vi "Get Joint Position.vi"(6 "JointType":T2 items=["SpineBase", "SpineMid", "Neck", "Head", "ShoulderLeft", "ElbowLeft", "WristLeft", "HandLeft", "ShoulderRight", "ElbowRight", "WristRight", "HandRight", "HipLeft", "KneeLeft", "AnkleLeft", "FootLeft", "HipRight", "KneeRight", "AnkleRight", "FootRight", "SpineShoulder", "HandTipLeft", "ThumbLeft", "HandTipRight", "ThumbRight"], 8 "error in (no error)":errorcluster, 9 "Coordinate Space":enum16{"Color Space", "Depth Space"}(ring), 10 "Joints":refnum<k24>, 11 "KinectSensor Reference":refnum<k24>) -> (0 "error out":errorcluster, 3 "Joint Position":T1 {"TrackingState" items=["NotTracked", "Inferred", "Tracked"]})   [LabVIEW 2014]
uses:
  Microsoft.Kinect
  controls/JointType.ctl
  controls/Joint Position.ctl
  Constants.vi
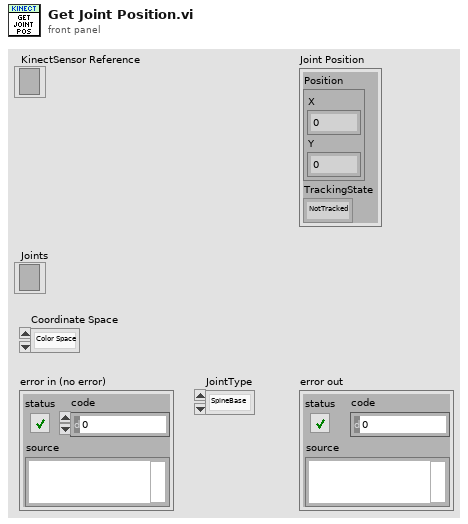
[diagram p1: front panel]
types:
  T1 = typedef "Joint Position.ctl" = cluster{"Position":cluster{"X":sgl, "Y":sgl}, "TrackingState":i32}
  T2 = typedef "JointType.ctl" = i32
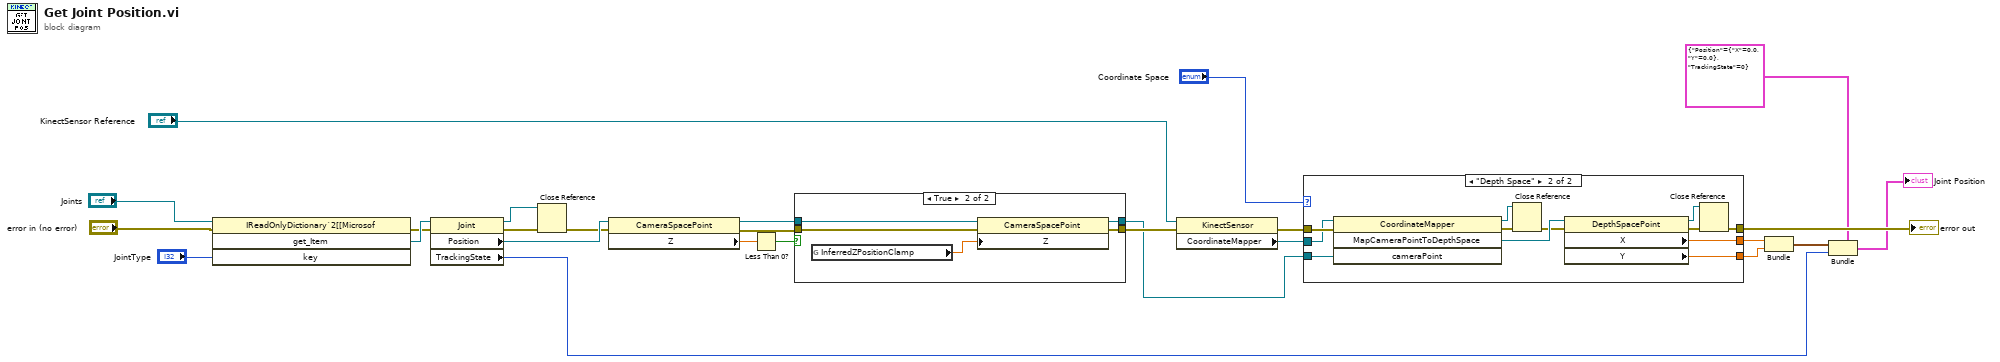
[diagram p0: block diagram]
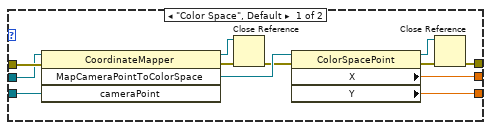
[diagram p2: hidden frame]
diagram:
  n1 = invoke class="IReadOnlyDictionary`2[[Microsof" method="get_Item"(reference="Joints", error in="error in (no error)", "key"="JointType") -> (error out=w13:errorcluster, "get_Item"=w14:refnum<k24>)  [unwired: 1 in, 2 out]
  n2 = property class="Joint"(reference=w14, error in=w13) -> (reference out=w8:refnum<k24>, error out=w9:errorcluster, "Position"=w12:refnum<k24>, "TrackingState"=w3:i32)
  n3 = Close Reference(reference=w8, error in (no error)=w9) -> (error out=w7:errorcluster)
  n4 = property class="CameraSpacePoint"(reference=w12, error in=w7) -> (reference out=w21:refnum<k24>, error out=w20:errorcluster, "Z"=w23:sgl)
  n5 = Less Than 0?(x=w23) -> (x < 0?=w22:bool)
  n6 = case shown="True" w22 {
    tunnel: w21 -> [w27 w32]
    tunnel: w20 -> [w28 w31]
    tunnel: [w28 w30] -> w19
    tunnel: [w27 w29] -> w18
    frame False {
    }
    frame True {
      n7 = global read "Constants.vi" "InferredZPositionClamp"() -> (w33:sgl)
      n8 = property class="CameraSpacePoint"(reference=w32, error in=w31, "Z"=w33) -> (reference out=w29:refnum<k24>, error out=w30:errorcluster)
    }
  }
  n9 = property class="KinectSensor"(reference="KinectSensor Reference", error in=w19) -> (error out=w26:errorcluster, "CoordinateMapper"=w25:refnum<k24>)  [unwired: 1 out]
  n10 = case shown="\"Depth Space\"" "Coordinate Space" {
    tunnel: w26 -> [w45 w57]
    tunnel: w25 -> [w44 w56]
    tunnel: w18 -> [w43 w55]
    tunnel: [w41 w53] -> w17
    tunnel: [w40 w52] -> w16
    tunnel: [w34 w46] -> w5
    frame "Color Space", Default {
      n11 = invoke class="CoordinateMapper" method="MapCameraPointToColorSpace"(reference=w44, error in=w45, "cameraPoint"=w43) -> (reference out=w37:refnum<k24>, error out=w39:errorcluster, "MapCameraPointToColorSpace"=w42:refnum<k24>)  [unwired: 1 in, 1 out]
      n12 = Close Reference(reference=w37, error in (no error)=w39) -> (error out=w38:errorcluster)
      n13 = property class="ColorSpacePoint"(reference=w42, error in=w38) -> (reference out=w35:refnum<k24>, error out=w36:errorcluster, "X"=w40:sgl, "Y"=w41:sgl)
      n14 = Close Reference(reference=w35, error in (no error)=w36) -> (error out=w34:errorcluster)
    }
    frame "Depth Space" {
      n15 = invoke class="CoordinateMapper" method="MapCameraPointToDepthSpace"(reference=w56, error in=w57, "cameraPoint"=w55) -> (reference out=w49:refnum<k24>, error out=w51:errorcluster, "MapCameraPointToDepthSpace"=w54:refnum<k24>)  [unwired: 1 in, 1 out]
      n16 = Close Reference(reference=w49, error in (no error)=w51) -> (error out=w50:errorcluster)
      n17 = property class="DepthSpacePoint"(reference=w54, error in=w50) -> (reference out=w47:refnum<k24>, error out=w48:errorcluster, "X"=w52:sgl, "Y"=w53:sgl)
      n18 = Close Reference(reference=w47, error in (no error)=w48) -> (error out=w46:errorcluster)
    }
  }
  "error out" <- w5
  n19 = Bundle("X"=w16, "Y"=w17) -> (w4:cluster{"X":sgl, "Y":sgl})  [unwired: 1 in]
  n20 = Bundle(cluster=T1 {"Position"={"X"=0.0, "Y"=0.0}, "TrackingState"=0} ("Joint Position"), "Position"=w4, "TrackingState"=w3) -> (→"Joint Position":T1)
